vi "lvEtherbone.VI-Tree.vi"   [LabVIEW 2009, in "lvEtherbone.lvlib"]
doc: "Contains all VIs of the LabVIEW-Etherbone interface.\n\nauthor: Dietrich Beck, GSI\nCopyright (C): GSI Helmholtzzentrum für Schwerionenforschung\nlicense: GPLv3\n\nFor details see description of lvEtherbone.lvlib"
uses:
  lvEtherbone.lvlib
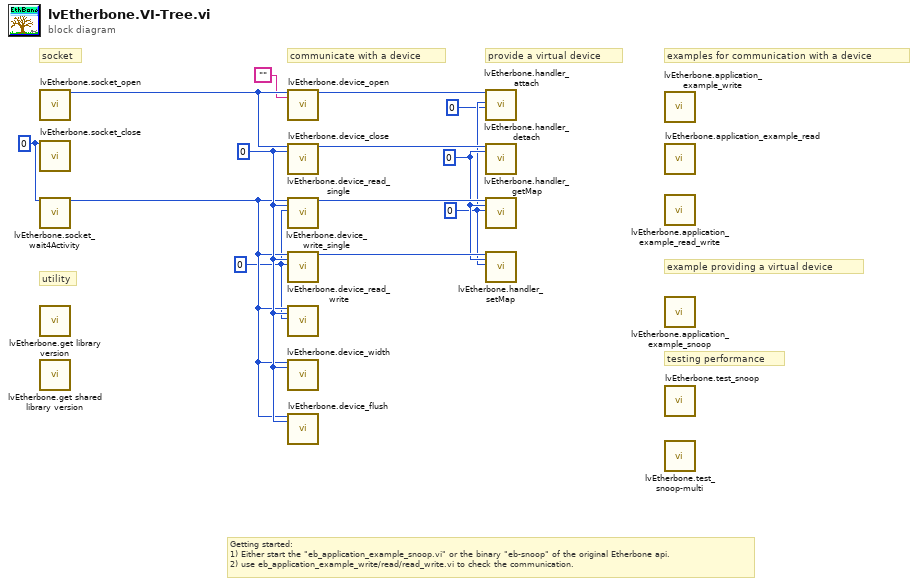
[diagram p0: block diagram]
diagram:
  w2 = u64 0 ("address")
  w3 = u64 0 ("address")
  w7 = 0 ("eb_socket_ID")
  w8 = 0 ("eb_handlerID")
  w9 = 0 ("eb_device_ID")
  # "utility"
  # "Getting started: \n1) Either start the \"eb_application_example_snoop.vi\" or the binary \"eb-snoop\" of the original Etherbone api.\n2) use eb_application_example_write/read/read_write.vi to check the communication."
  # "testing performance"
  # "example providing a virtual device"
  # "examples for communication with a device"
  # "provide a virtual device"
  # "communicate with a device"
  # "socket"
  n1 = call "lvEtherbone.socket_open.vi"() -> ("eb_socket_ID"=w6:i32)  [unwired: 17 in, 2 out]
  n2 = call "lvEtherbone.socket_close.vi"("eb_socket_ID"=w7) -> ()  [unwired: 17 in, 2 out]
  n3 = call "lvEtherbone.socket_wait4Activity.vi"("eb_socketID"=w7) -> ("eb_socketID out"=w5:i32)  [unwired: 12 in, 6 out]
  n4 = call "lvEtherbone.get library version.vi"() -> ()  [unwired: 1 in, 1 out]
  n5 = call "lvEtherbone.get shared library version.vi"() -> ()  [unwired: 17 in, 3 out]
  n6 = call "lvEtherbone.device_open.vi"("eb_socket_ID"=w6, "ip_port"="") -> ("eb_socket_ID out"=w13:i32)  [unwired: 13 in, 4 out]
  n7 = call "lvEtherbone.device_close.vi"("eb_socket_ID"=w6, "eb_device_ID"=w9) -> ("eb_socket_ID out"=w12:i32)  [unwired: 15 in, 2 out]
  n8 = call "lvEtherbone.device_read_single.vi"("eb_socket_ID"=w5, "eb_device_ID"=w9, "address"=w3) -> ("eb_socket_ID out"=w11:i32)  [unwired: 11 in, 5 out]
  n9 = call "lvEtherbone.device_write_single.vi"("eb_socketID"=w5, "eb_deviceID"=w9, "address"=w3) -> ("eb_socketID out"=w10:i32)  [unwired: 13 in, 3 out]
  n10 = call "lvEtherbone.device_read_write.vi"("eb_socket_ID"=w5, "eb_device_ID"=w9, "addressR"=w3) -> ()  [unwired: 11 in, 6 out]
  n11 = call "lvEtherbone.device_width.vi"("eb_socket_ID"=w5, "eb_device_ID"=w9) -> ()  [unwired: 13 in, 5 out]
  n12 = call "lvEtherbone.device_flush.vi"("eb_socket_ID"=w5, "eb_device_ID"=w9) -> ()  [unwired: 15 in, 3 out]
  n13 = call "lvEtherbone.handler_attach.vi"("eb_socket_ID"=w13, "baseAddress"=w2, "maskAddress"=0) -> ()  [unwired: 13 in, 4 out]
  n14 = call "lvEtherbone.handler_detach.vi"("eb_socketID"=w12, "eb_handlerID"=w8) -> ()  [unwired: 15 in, 3 out]
  n15 = call "lvEtherbone.handler_getMap.vi"("eb_socket_ID"=w11, "eb_handlerID"=w8, "address"=w2) -> ()  [unwired: 12 in, 5 out]
  n16 = call "lvEtherbone.handler_setMap.vi"("eb_socketID"=w10, "eb_handlerID"=w8, "address"=w2) -> ()  [unwired: 13 in, 4 out]
  n17 = call "lvEtherbone.application_example_write.vi"() -> ()  [unwired: 12 in]
  n18 = call "lvEtherbone.application_example_read.vi"() -> ()  [unwired: 1 in]
  n19 = call "lvEtherbone.application_example_read_write.vi"() -> ()  [unwired: 1 in]
  n20 = call "lvEtherbone.application_example_snoop.vi"() -> ()  [unwired: 12 in]
  n21 = call "lvEtherbone.test_snoop.vi"() -> ()  [unwired: 1 in]
  n22 = call "lvEtherbone.test_snoop-multi.vi"() -> ()  [unwired: 1 in]
